vi "VI_Heat_Tape_Final_subVI.vi"(0 "VISA Refnum in":refnum<visa-resource-name>, 1 "in":bool, 2 "WFChart Refnum 2":refnum<vi>, 3 "Slide Refnum 2":refnum<vi>, 4 "COM Port (Station 02)":refnum<visa-resource-name>, 5 "WFChart Refnum":refnum<vi>, 6 "Slide Refnum":refnum<vi>, 7 "error in (no error)":errorcluster, 8 "Hysterisis (Station 02)":string, 9 "error check":errorcluster, 10 "Set Value (Station 02)":string, 12 "Set Value (Station 01)":string, 14 "Hysterisis (Station 01)":string) -> (13 "Register and RAW value 2":u16[](array[numeric]), 15 "Connection (Station 02)":bool, 16 "Connection Status (Station 01)":bool, 17 "Query Message":string, 18 "Register and RAW value":u16[](array[numeric]), 19 "Query Message 2":string, 20 "Value 3":sgl, 21 "Heat Tape Temperature Profiles (ºF)":dbl(slide) scale=60.0..80.0, 22 "Current Temperature (ºF)":string, 23 "out":cluster{dbl, dbl, dbl, dbl}(graph), 24 "Value 4":sgl, 25 "?":cluster{dbl, dbl}(graph), 26 "Current Temperature (ºF) 2":string, 27 "Heat Tape 01  Temperature (ºF) 2":dbl(slide) scale=61.0..81.0)   [LabVIEW 2019]
uses:
  <vilib>/NI/Modbus Library/API/Wrapper/Create Serial Master.vi
  <vilib>/NI/Modbus Library/API/Master/Modbus Master.lvclass
  <vilib>/NI/Modbus Library/API/Wrapper/API Main.lvlib
  <vilib>/NI/Modbus Library/Transmission Data Unit/RTU/RTU Data Unit.lvclass
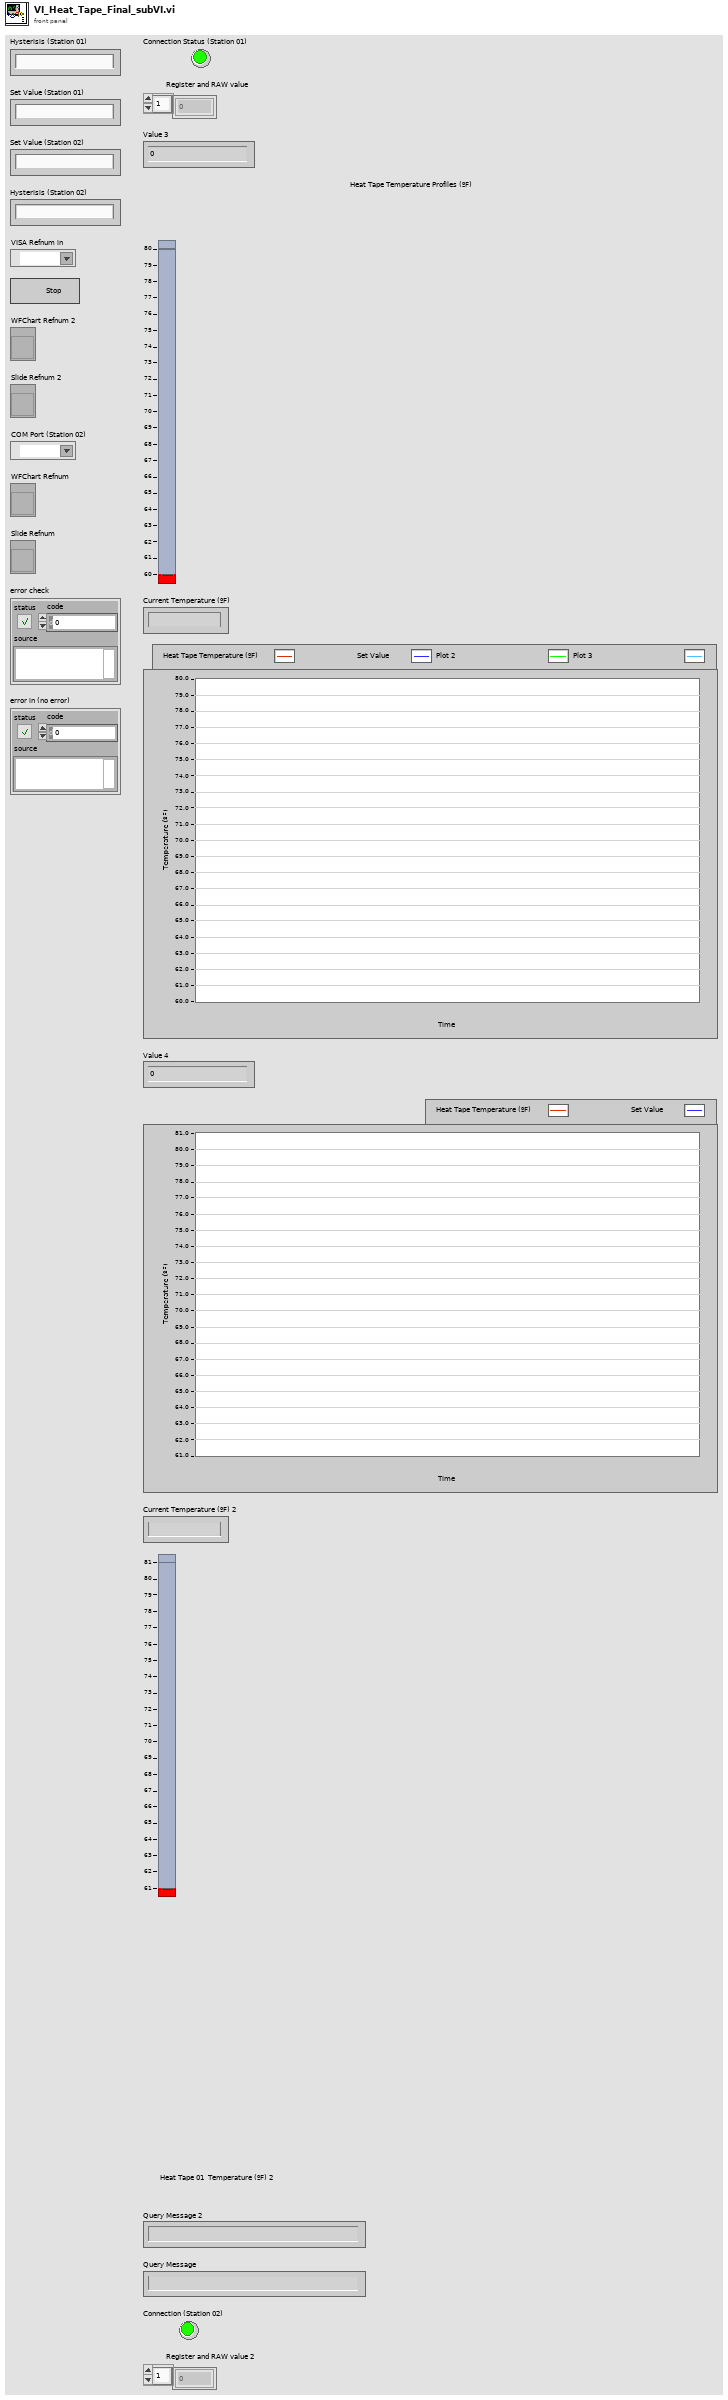
[diagram p1: front panel]
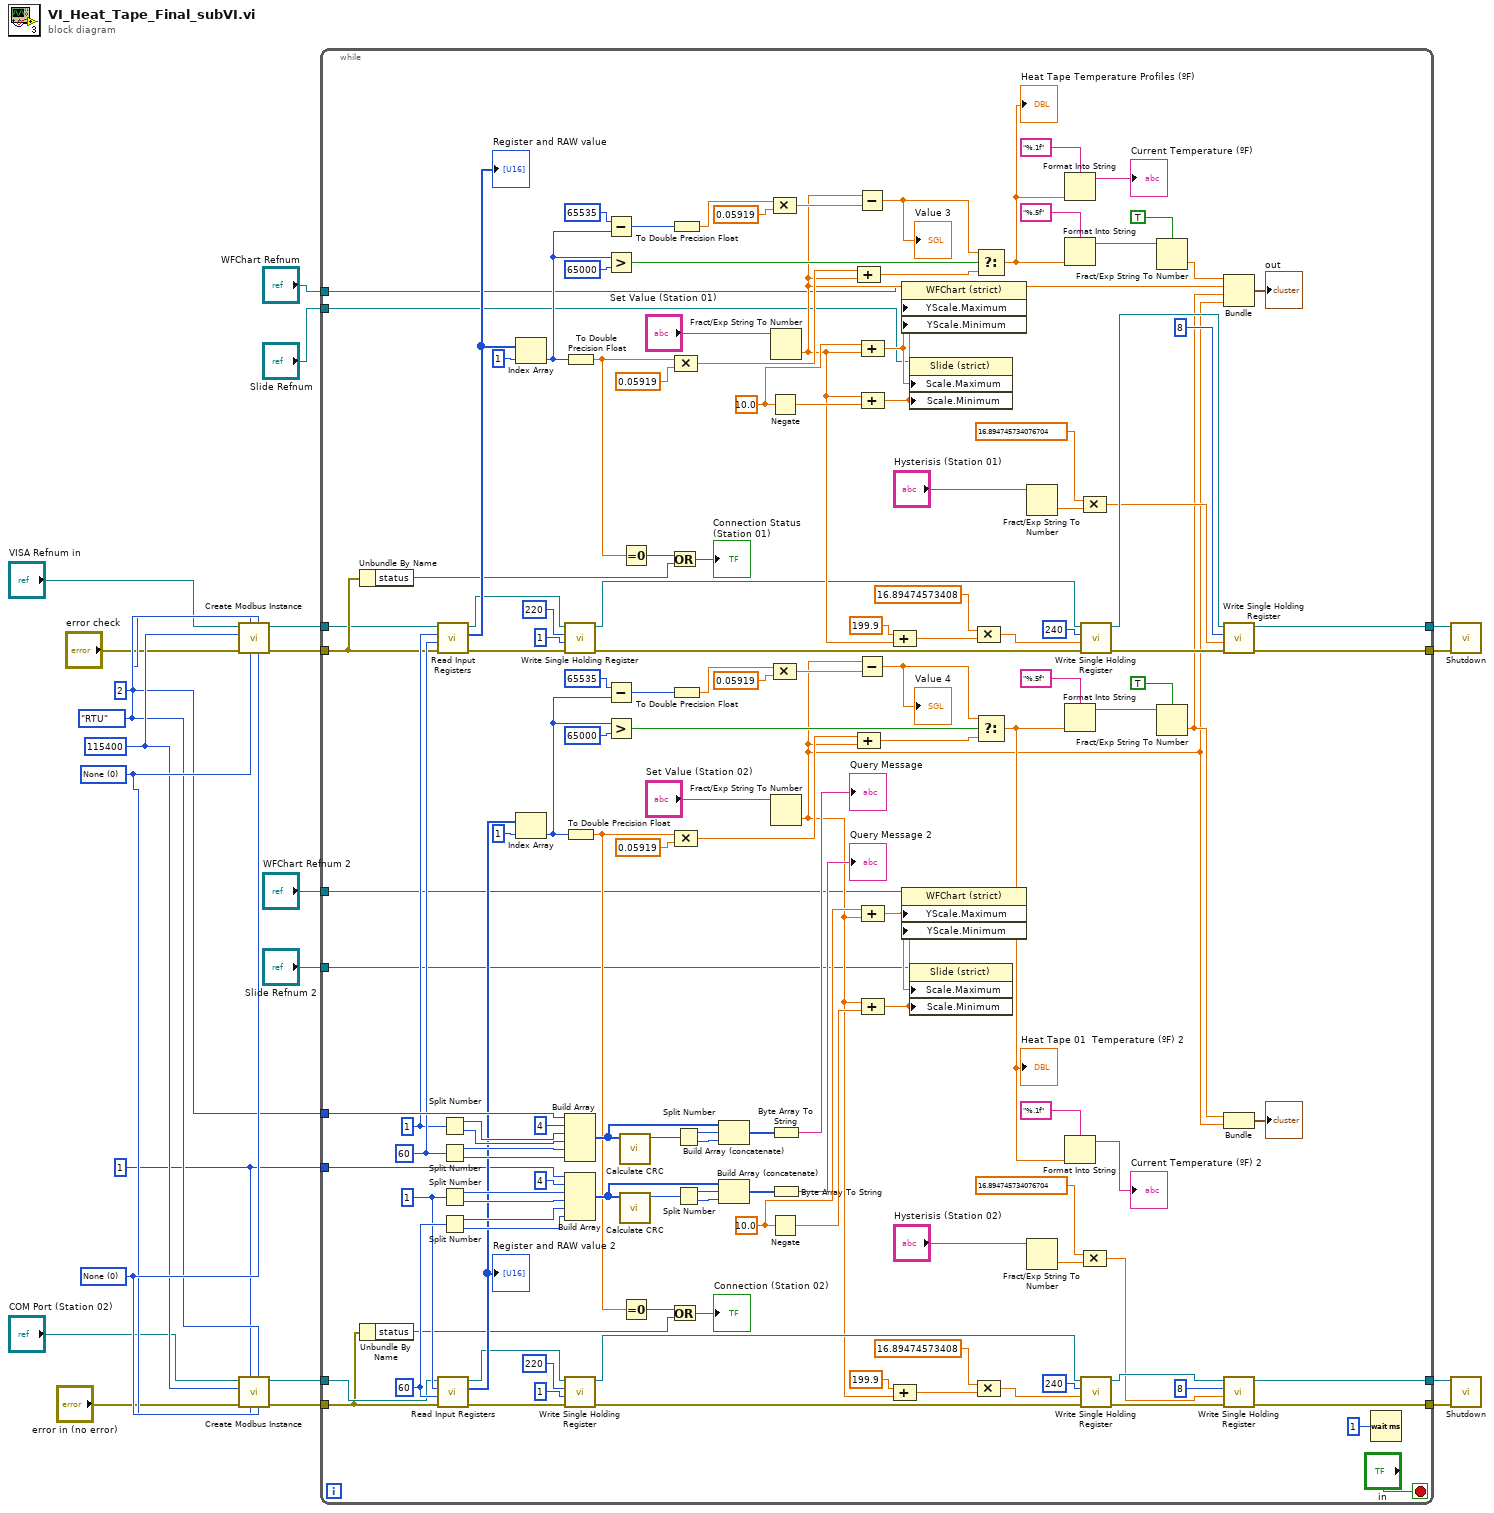
[diagram p0: block diagram]
diagram:
  w18 = u8 1 ("unit ID (Defaut: 1)")
  w9 = u8 2 ("unit ID (Defaut: 1)")
  w19 = enum16{"RTU", "ASCII"}."RTU" ("Serial Type (Default: RTU)")
  w20 = u32 115400 ("Baud Rate (Default: 115400)")
  w22 = u16 0 items=["None", "XON/XOFF", "RTS/CTS", "XON/XOFF & RTS/CTS", "DTR/DSR", "XON/XOFF & DTR/DSR"] ("Flow Control (Default: None)")
  w21 = u16 0 items=["None", "Odd", "Even", "Mark", "Space"] ("Parity (Default: None)")
  n1 = call-poly <vilib>:"Create Modbus Instance.vi"("flow control (none)"=w22, "serial type"=w19, "parity (even)"=w21, "unit ID"=w9, "error in"="error check", "baud rate"=w20, "VISA resource name"="VISA Refnum in") -> ("error out"=w7:errorcluster, "serial master instance"=w6:refnum<class "Modbus Master.lvclass">)  [unwired: 3 in]
  n2 = call-poly <vilib>:"Create Modbus Instance.vi"("flow control (none)"=w22, "serial type"=w19, "parity (even)"=w21, "unit ID"=w18, "error in"="error in (no error)", "baud rate"=w20, "VISA resource name"="COM Port (Station 02)") -> ("error out"=w15:errorcluster, "serial master instance"=w16:refnum<class "Modbus Master.lvclass">)  [unwired: 3 in]
  n3 = while {
    tunnel: w6 -> [w131]
    tunnel: w7 -> [w139]
    tunnel: w9 -> [w164]
    tunnel: [w105] -> w10
    tunnel: [w104] -> w11
    tunnel: [w33] -> w12
    tunnel: [w32] -> w13
    tunnel: w15 -> [w30]
    tunnel: w16 -> [w31]
    tunnel: w18 -> [w29]
    tunnel: "Slide Refnum" -> [w26]
    tunnel: "WFChart Refnum" -> [w25]
    tunnel: "Slide Refnum 2" -> [w24]
    tunnel: "WFChart Refnum 2" -> [w23]
    stop <- "in" stop-if-true
    w82 = u16 1 ("starting address (Default: 1)")
    w83 = u16 60 ("number of inputs (Defaut: 60)")
    w60 = 10.0 ("value")
    w150 = u16 1 ("starting address (Default: 1)")
    w151 = u16 60 ("number of inputs (Defaut: 60)")
    w124 = 10.0 ("value")
    n4 = Unbundle By Name(w139) -> ("status"=w136:bool)
    n5 = Unbundle By Name(w30) -> ("status"=w70:bool)
    n6 = call-dynamic "Read Input Registers.vi"("error in"=w139, "number of inputs"=w151, "starting address"=w150, "Modbus master in"=w131) -> ("error out"=w108:errorcluster, "register values"=w148:u16[], "Modbus master out"=w109:refnum<class "Modbus Master.lvclass">)  [unwired: 5 in]
    "Register and RAW value" <- w148
    n7 = call-dynamic "Read Input Registers.vi"("error in"=w30, "number of inputs"=w83, "starting address"=w82, "Modbus master in"=w31) -> ("error out"=w44:errorcluster, "register values"=w81:u16[], "Modbus master out"=w45:refnum<class "Modbus Master.lvclass">)  [unwired: 5 in]
    "Register and RAW value 2" <- w81
    n8 = Split Number(x=w150) -> (hi(x)=w156:u8, lo(x)=w155:u8)
    n9 = Split Number(x=w151) -> (hi(x)=w154:u8, lo(x)=w153:u8)
    n10 = Split Number(x=w82) -> (hi(x)=w87:u8, lo(x)=w86:u8)
    n11 = Split Number(x=w83) -> (hi(x)=w85:u8, lo(x)=w84:u8)
    n12 = Index Array(array=w148, index=1) -> (element=w125:u16)
    n13 = Index Array(array=w81, index=1) -> (element=w61:u16)
    n14 = call-dynamic "Write Single Holding Register.vi"("error in"=w108, "register to write"=u16 1, "address"=u16 220, "Modbus master in"=w109) -> ("error out"=w102:errorcluster, "Modbus master out"=w103:refnum<class "Modbus Master.lvclass">)  [unwired: 6 in]
    n15 = Build Array(w164, u8 4 ("element"), w156, w155, w154, w153) -> (w162:u8[])
    n16 = Build Array(w29, u8 4 ("element"), w87, w86, w85, w84) -> (w93:u8[])
    n17 = call-dynamic "Write Single Holding Register.vi"("error in"=w44, "register to write"=u16 1, "address"=u16 220, "Modbus master in"=w45) -> ("error out"=w41:errorcluster, "Modbus master out"=w42:refnum<class "Modbus Master.lvclass">)  [unwired: 6 in]
    n18 = To Double Precision Float(number=w125) -> (double precision float=w138:dbl)
    n19 = To Double Precision Float(number=w61) -> (double precision float=w72:dbl)
    n20 = Subtract(x=u16 65535 ("y"), y=w125) -> (x-y=w117:u16)
    n21 = Greater?(x=w125, y=u16 65000) -> (0:w113:bool)
    n22 = Subtract(x=u16 65535 ("y"), y=w61) -> (x-y=w53:u16)
    n23 = Greater?(x=w61, y=u16 65000) -> (0:w49:bool)
    n24 = call <vilib>:"Calculate CRC.vi"("data"=w162) -> ("CRC-16"=w161:u16)  [unwired: 10 in]
    n25 = call <vilib>:"Calculate CRC.vi"("data"=w93) -> ("CRC-16"=w92:u16)  [unwired: 10 in]
    n26 = Equal To 0?(x=w138) -> (x = 0?=w135:bool)
    n27 = Equal To 0?(x=w72) -> (x = 0?=w69:bool)
    n28 = Or(x=w135, y=w136) -> (x .or. y?=→"Connection Status (Station 01)":bool)
    n29 = Or(x=w69, y=w70) -> (x .or. y?=→"Connection (Station 02)":bool)
    n30 = To Double Precision Float(number=w117) -> (double precision float=w119:dbl)
    n31 = To Double Precision Float(number=w53) -> (double precision float=w55:dbl)
    n32 = Split Number(x=w161) -> (hi(x)=w160:u8, lo(x)=w159:u8)
    n33 = Split Number(x=w92) -> (hi(x)=w91:u8, lo(x)=w90:u8)
    n34 = Compound Arithmetic op=MULTIPLY(w138, 0.05919 ("value")) -> (w146:dbl)
    n35 = Compound Arithmetic op=MULTIPLY(w72, 0.05919 ("value")) -> (w79:dbl)
    n36 = Build Array (concatenate)(w162, w160, w159) -> (w158:u8[])
    n37 = Build Array (concatenate)(w93, w91, w90) -> (w89:u8[])
    n38 = Negate(x=w124) -> (-x=w123:dbl)
    n39 = Negate(x=w60) -> (-x=w59:dbl)
    n40 = Fract/Exp String To Number(string="Set Value (Station 01)") -> (number=w107:dbl)  [unwired: 3 in, 1 out]
    n41 = Fract/Exp String To Number(string="Set Value (Station 02)") -> (number=w27:dbl)  [unwired: 3 in, 1 out]
    n42 = Byte Array To String(unsigned byte array=w158) -> (string=→"Query Message":string)
    n43 = Byte Array To String(unsigned byte array=w89) -> (string=→"Query Message 2":string)
    n44 = Compound Arithmetic op=MULTIPLY(w119, 0.05919 ("value")) -> (w116:dbl)
    n45 = Compound Arithmetic op=MULTIPLY(w55, 0.05919 ("value")) -> (w52:dbl)
    n46 = Subtract(x=w107, y=w116) -> (x-y=w115:dbl)
    "Value 3" <- w115
    n47 = Subtract(x=w27, y=w52) -> (x-y=w51:dbl)
    "Value 4" <- w51
    n48 = Compound Arithmetic op=ADD(w146, w107) -> (w114:dbl)
    n49 = Compound Arithmetic op=ADD(w79, w27) -> (w50:dbl)
    n50 = Compound Arithmetic op=ADD(w124, w107) -> (w122:dbl)
    n51 = Compound Arithmetic op=ADD(w107, w123) -> (w121:dbl)
    n52 = Compound Arithmetic op=ADD(w60, w27) -> (w58:dbl)
    n53 = Compound Arithmetic op=ADD(w27, w59) -> (w57:dbl)
    n54 = Compound Arithmetic op=ADD(199.9 ("value"), w107) -> (w129:dbl)
    n55 = Compound Arithmetic op=ADD(199.9 ("value"), w27) -> (w65:dbl)
    n56 = property on="Property Node" class="WFChart (strict)"(reference=w25, "YScale.Maximum"=w122, "YScale.Minimum"=w121) -> ()  [unwired: 1 in, 2 out]
    n57 = property on="Property Node" class="WFChart (strict)"(reference=w23, "YScale.Maximum"=w58, "YScale.Minimum"=w57) -> ()  [unwired: 1 in, 2 out]
    n58 = property on="Property Node" class="Slide (strict)"(reference=w26, "Scale.Maximum"=w122, "Scale.Minimum"=w121) -> ()  [unwired: 1 in, 2 out]
    n59 = property on="Property Node" class="Slide (strict)"(reference=w24, "Scale.Maximum"=w58, "Scale.Minimum"=w57) -> ()  [unwired: 1 in, 2 out]
    n60 = Select(t=w115, s=w113, f=w114) -> (s? t:f=w120:dbl)
    "Heat Tape Temperature Profiles (ºF)" <- w120
    n61 = Select(t=w51, s=w49, f=w50) -> (s? t:f=w56:dbl)
    "Heat Tape 01  Temperature (ºF) 2" <- w56
    n62 = Compound Arithmetic op=MULTIPLY(16.89474573408 ("value"), w129) -> (w99:dbl)
    n63 = Compound Arithmetic op=MULTIPLY(16.89474573408 ("value"), w65) -> (w38:dbl)
    n64 = Fract/Exp String To Number(string="Hysterisis (Station 01)") -> (number=w97:dbl)  [unwired: 3 in, 1 out]
    n65 = Fract/Exp String To Number(string="Hysterisis (Station 02)") -> (number=w36:dbl)  [unwired: 3 in, 1 out]
    n66 = Format Into String(format string="%.1f", w120) -> (resulting string=→"Current Temperature (ºF)":string)  [unwired: 2 in, 1 out]
    n67 = Format Into String(format string="%.5f", w120) -> (resulting string=w141:string)  [unwired: 2 in, 1 out]
    n68 = Format Into String(format string="%.5f", w56) -> (resulting string=w74:string)  [unwired: 2 in, 1 out]
    n69 = Format Into String(format string="%.1f", w56) -> (resulting string=→"Current Temperature (ºF) 2":string)  [unwired: 2 in, 1 out]
    n70 = call-dynamic "Write Single Holding Register.vi"("error in"=w102, "register to write"=w99, "address"=u16 240, "Modbus master in"=w103) -> ("error out"=w101:errorcluster, "Modbus master out"=w100:refnum<class "Modbus Master.lvclass">)  [unwired: 6 in]
    n71 = call-dynamic "Write Single Holding Register.vi"("error in"=w41, "register to write"=w38, "address"=u16 240, "Modbus master in"=w42) -> ("error out"=w40:errorcluster, "Modbus master out"=w39:refnum<class "Modbus Master.lvclass">)  [unwired: 6 in]
    n72 = Compound Arithmetic op=MULTIPLY(16.894745734076704 ("value"), w97) -> (w96:dbl)
    n73 = Compound Arithmetic op=MULTIPLY(16.894745734076704 ("value"), w36) -> (w35:dbl)
    n74 = Fract/Exp String To Number(use system decimal point (T)=TRUE, string=w141) -> (number=w134:dbl)  [unwired: 2 in, 1 out]
    n75 = Fract/Exp String To Number(use system decimal point (T)=TRUE, string=w74) -> (number=w28:dbl)  [unwired: 2 in, 1 out]
    n76 = Bundle(w134, w107, w28, w27) -> (→"out":cluster{dbl, dbl, dbl, dbl})  [unwired: 1 in]
    n77 = call-dynamic "Write Single Holding Register.vi"("error in"=w101, "register to write"=w96, "address"=u16 8, "Modbus master in"=w100) -> ("error out"=w104:errorcluster, "Modbus master out"=w105:refnum<class "Modbus Master.lvclass">)  [unwired: 6 in]
    n78 = Bundle(w28, w27) -> (→"?":cluster{dbl, dbl})  [unwired: 1 in]
    n79 = call-dynamic "Write Single Holding Register.vi"("error in"=w40, "register to write"=w35, "address"=u16 8, "Modbus master in"=w39) -> ("error out"=w32:errorcluster, "Modbus master out"=w33:refnum<class "Modbus Master.lvclass">)  [unwired: 6 in]
    n80 = Wait (ms)(milliseconds to wait=u32 1) -> ()  [unwired: 1 out]
  }
  n81 = call-dynamic "Shutdown.vi"("error in"=w11, "Modbus master in"=w10) -> ()  [unwired: 9 in, 1 out]
  n82 = call-dynamic "Shutdown.vi"("error in"=w13, "Modbus master in"=w12) -> ()  [unwired: 9 in, 1 out]
